vi "AutoStates.vi"(6 "WasHot?":bool, 8 "error in (no error)":errorcluster, 9 "SwitchToLowGear?":bool, 10 "AutoMode":T1, 11 "AutoState":T2) -> (0 "error out":errorcluster, 4 "Hot?":bool)   [LabVIEW 2013]
uses:
  AutoStates.ctl
  AutoMode.ctl
  DoubleSolenoidAction.ctl
  SingleSolenoidAction.ctl
  ServoAction.ctl
  RollerAction.ctl
  CollectorWrapAction.ctl
  SonarAction.ctl
  AutoAlignMode.ctl
  TankDriveAction.ctl
  ShooterWrapperAction.ctl
panel:
  out "ElapsedTime":u32
  in  "RotateWait":u32=300
  in  "RotateMotorInput":dbl=0.7
  out "RaiseArmTimedOut":bool
  in  "CollectorArmSpeed":dbl=1.0 format="%#_13g"
  in  "RaiseArmTimeout":u32=800
  in  "LowerArmTimeout":u32=800
  in  "PreRaiseArmWait":u32=500
  in  "PreShootWait":u32
  in  "StartShootTime":u32=4500
  out "DriveTimeOut":bool
  in  "MaxMotorChangeBackward":dbl=0.025
  in  "MaxMotorChangeForward":dbl=0.05
  in  "DefaultMotorInput":dbl=0.7
  in  "SlowdownDistance":dbl=24.0 format="%#_13g"
  in  "BrakeDistance":dbl=6.0 format="%#_13g"
  in  "FarShotDistance":dbl=150.0 format="%#_13g"
  in  "CloseShotDistance":dbl=36.0 format="%#_13g"
  in  "FarShotMinTime":u32=1000
  in  "CloseShotMinTime":u32=2000
  in  "FarShotTimeout":u32=4000
  in  "CloseShotTimeout":u32=4000
  in  "RaiseServoAngle":i32=100
  out "LowerArmTimedOut":bool
  in  "PreCollectWait":u32=400
  out "HotGoalTimedOut?":bool
  in  "CheckHotGoalTimeout":u32=1000
  in  "ServoInitAngle":i32=140
  # "ARM"
  # "HOT GOAL"
  # "SERVO"
  # "OUTPUT"
  # "SHOOT"
  # "ROTATE"
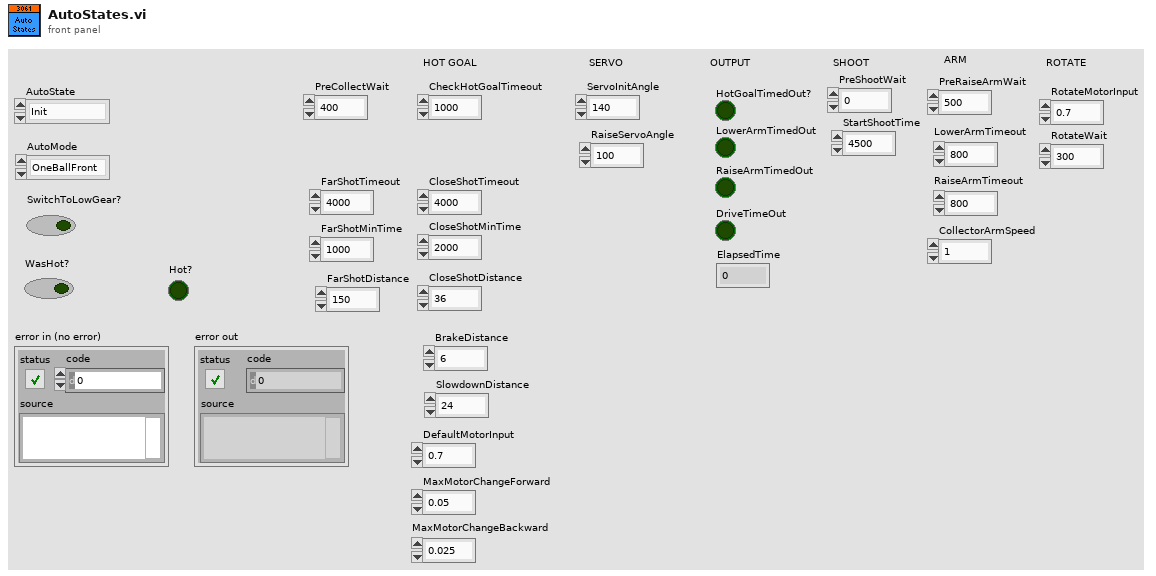
[diagram p1: front panel]
types:
  T1 = typedef "AutoMode.ctl" = enum16{"OneBallFront", "OneBallCollector", "TwoBallNormal", "TwoBallHot"}
  T2 = typedef "AutoStates.ctl" = enum16{"Init", "LowerArm", "CheckGoal", "Collect", "StopCollect", "RaiseServo", "Drive", "Wait", "ShootCollectorUp", "RaiseArm", "ShootCollectorDown", "Rotate1", "Rotate2", "Stop"}
  T3 = typedef "ServoAction.ctl" = enum16{"Init", "SetAngle", "GetAngle", "Lower", "Raise", "Disable"}
  T4 = typedef "DoubleSolenoidAction.ctl" = enum16{"Init", "Middle", "In", "Out"}
  T5 = typedef "SingleSolenoidAction.ctl" = enum16{"Init", "SetState", "Disable"}
  T6 = typedef "RollerAction.ctl" = enum16{"Init", "Off", "Forward", "Reverse"}
  T7 = typedef "CollectorWrapAction.ctl" = enum16{"PreCollect", "Collect", "Stop"}
  T8 = typedef "TankDriveAction.ctl" = enum16{"Init", "LinearDrive", "SetValue", "Disable"}
  T9 = typedef "AutoAlignMode.ctl" = enum16{"Fullspeed", "Linear"}
  T10 = typedef "SonarAction.ctl" = enum16{"Init", "ReadValue", "Disable"}
  T11 = typedef "ShooterWrapperAction.ctl" = enum16{"Init", "CollectorDown", "CollectorUp"}
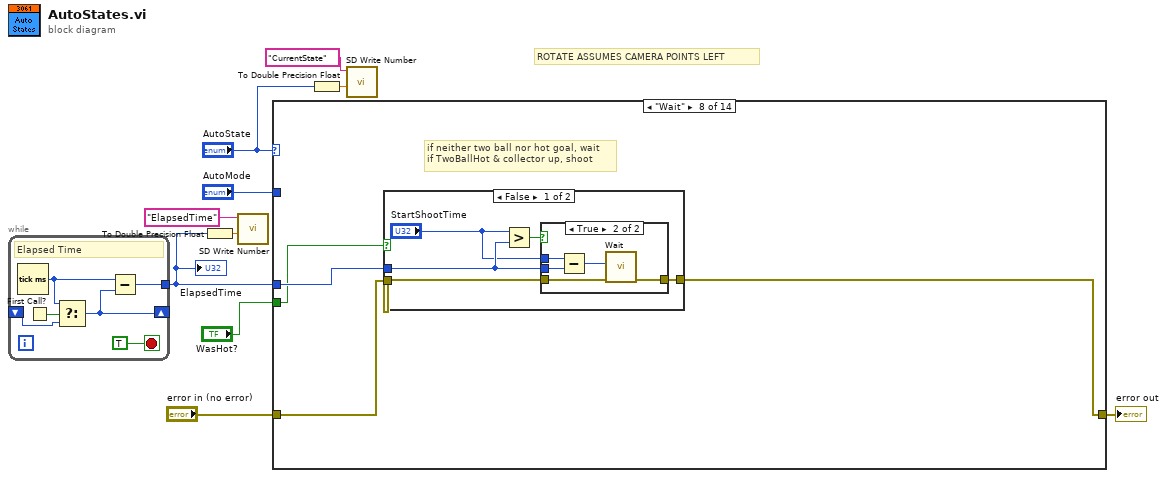
[diagram p0: block diagram]
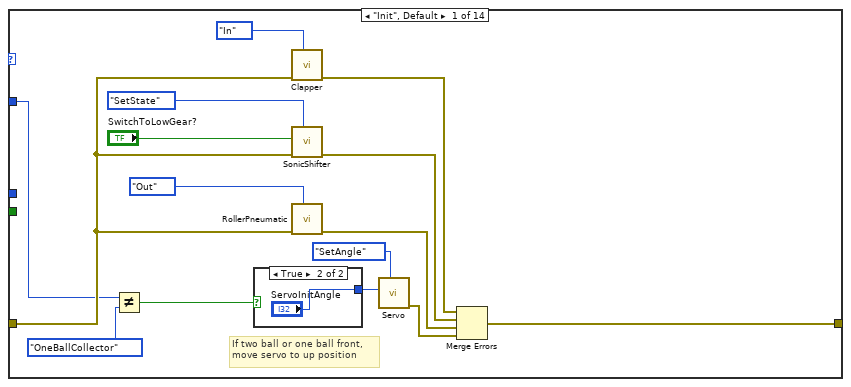
[diagram p2: hidden frame]
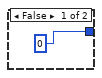
[diagram p3: hidden frame]
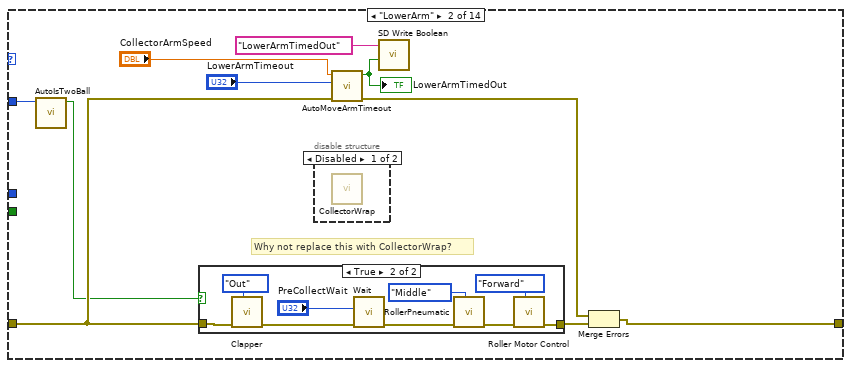
[diagram p4: hidden frame]
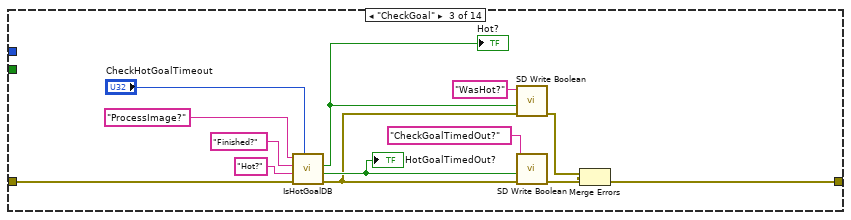
[diagram p7: hidden frame]
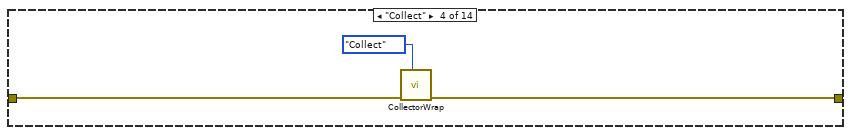
[diagram p8: hidden frame]
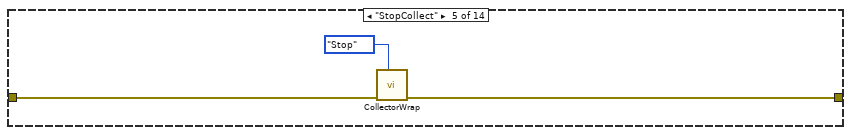
[diagram p9: hidden frame]
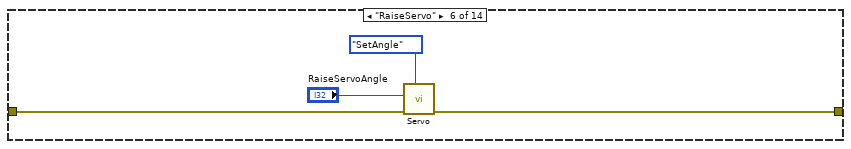
[diagram p10: hidden frame]
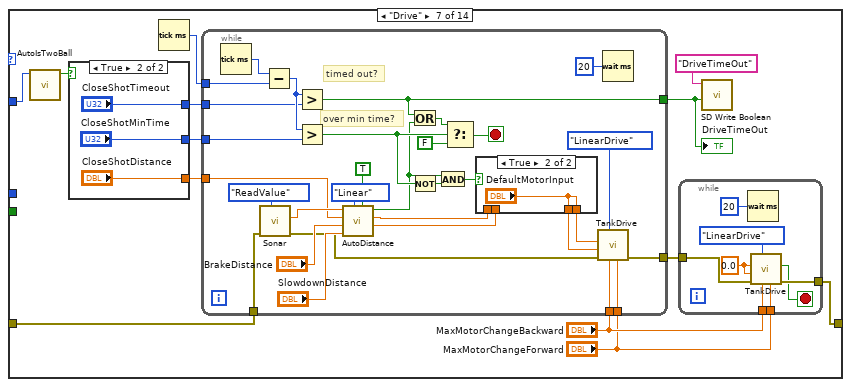
[diagram p11: hidden frame]
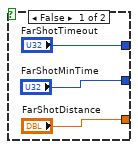
[diagram p13: hidden frame]
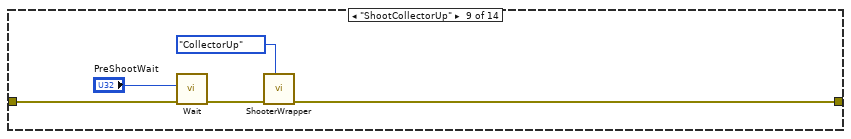
[diagram p16: hidden frame]
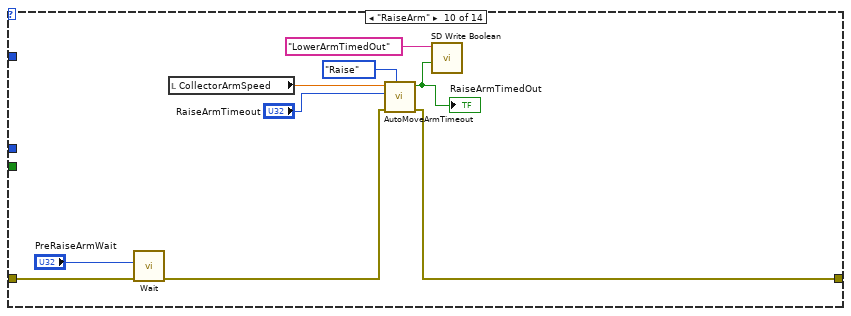
[diagram p17: hidden frame]
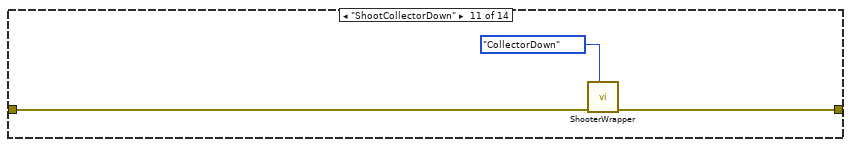
[diagram p18: hidden frame]
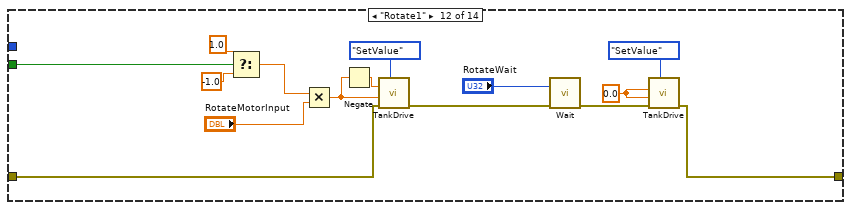
[diagram p19: hidden frame]
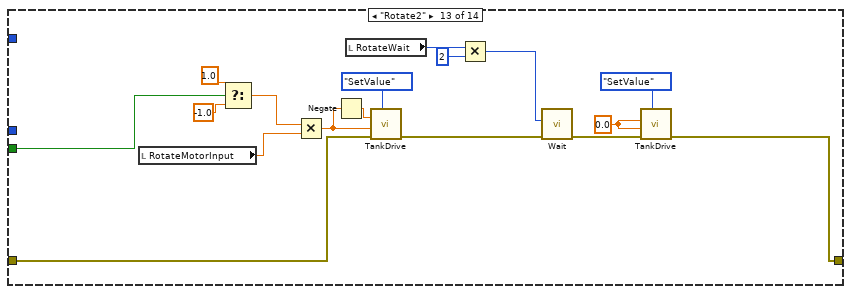
[diagram p20: hidden frame]
diagram:
  # "ROTATE ASSUMES CAMERA POINTS LEFT"
  n1 = while {
    shift-right: [w12] -> _
    shift-left: _ -> [w14]
    tunnel: [w11] -> w1
    stop <- TRUE stop-if-true
    # "Elapsed Time"
    n2 = Tick Count (ms)() -> (millisecond timer value=w13:u32)
    n3 = First Call?() -> (First Call?: T/F=w16:bool)
    n4 = Select(t=w13, s=w16, f=w14) -> (s? t:f=w12:u32)
    n5 = Subtract(x=w13, y=w12) -> (x-y=w11:u32)
  }
  "ElapsedTime" <- w1
  n6 = To Double Precision Float(number=w1) -> (double precision float=w2:dbl)
  n7 = call <vilib>:"SD Write Number.vi"("Numeric"=w2, "Name"="ElapsedTime") -> ()  [unwired: 8 in, 2 out]
  n8 = case shown="\"Wait\"" "AutoState" {
    tunnel: "AutoMode" -> [w26 w37 _ _ _ _ w89 _ _ _ _ _ _ _]
    tunnel: [w28 w41 w55 w67 w70 w74 w78 w139 w154 w161 w170 w171 w187 w203] -> w8
    tunnel: "error in (no error)" -> [w27 w42 w61 w68 w71 w73 w83 w140 w158 w166 w168 w172 w186 w204]
    tunnel: w1 -> [_ _ _ _ _ _ _ w141 _ _ _ _ _ _]
    tunnel: "WasHot?" -> [_ _ _ _ _ _ _ w138 _ _ _ w173 w188 _]
    frame "Init", Default {
      # "If two ball or one ball front, \nmove servo to up position"
      n9 = Not Equal?(x=w26, y=AutoMode."OneBallCollector") -> (x != y?=w18:bool)
      n10 = case shown="True" w18 {
        tunnel: [0 "ServoInitAngle"] -> w24
        frame False {
        }
        frame True {
        }
      }
      n11 = call "Clapper.vi"("State"=DoubleSolenoidAction."In", "Error in"=w27) -> ("Error out"=w19:errorcluster)  [unwired: 9 in]
      n12 = call "SonicShifter.vi"("Action"=SingleSolenoidAction."SetState", "error in (no error)"=w27, "Actuate?"="SwitchToLowGear?") -> ("error out"=w20:errorcluster)  [unwired: 8 in]
      n13 = call "RollerPneumatic.vi"("State"=DoubleSolenoidAction."Out", "Error in"=w27) -> ("Error out"=w21:errorcluster)  [unwired: 9 in]
      n14 = call "Servo.vi"("Action"=ServoAction."SetAngle", "Angle (deg)"=w24) -> ("error out"=w22:errorcluster)  [unwired: 8 in, 1 out]
      n15 = Merge Errors(w19, w20, w21, w22) -> (w28:errorcluster)
    }
    frame "LowerArm" {
      # "Why not replace this with CollectorWrap?"
      n16 = call "AutoIsTwoBall.vi"("AutoMode"=w37) -> ("IsTwoBall?"=w36:bool)  [unwired: 10 in]
      n17 = case shown="True" w36 {
        tunnel: [w44 w47] -> w40
        tunnel: w42 -> [w44 w48]
        frame False {
        }
        frame True {
          n18 = call "Clapper.vi"("State"=DoubleSolenoidAction."Out", "Error in"=w48) -> ("Error out"=w52:errorcluster)  [unwired: 9 in]
          n19 = call "Wait.vi"("error in"=w52, "milliseconds to wait"="PreCollectWait") -> ("error out"=w50:errorcluster)  [unwired: 9 in]
          n20 = call "RollerPneumatic.vi"("State"=DoubleSolenoidAction."Middle", "Error in"=w50) -> ("Error out"=w53:errorcluster)  [unwired: 9 in]
          n21 = call "Roller Motor Control.vi"("Action"=RollerAction."Forward", "Error in"=w53) -> ("Error out"=w47:errorcluster)  [unwired: 9 in]
        }
      }
      n22 = disable-structure shown="Disabled" {
        frame Disabled {
          n23 = call "CollectorWrap.vi"() -> ()  [unwired: 11 in, 1 out]
        }
        frame Enabled {
        }
      }
      n24 = call "AutoMoveArmTimeout.vi"("error in (no error)"=w42, "Timeout"="LowerArmTimeout", "CollectorArmSpeed"="CollectorArmSpeed") -> ("error out"=w39:errorcluster, "TimedOut?"=w38:bool)  [unwired: 7 in]
      "LowerArmTimedOut" <- w38
      n25 = call <vilib>:"SD Write Boolean.vi"("Boolean"=w38, "Name"="LowerArmTimedOut") -> ()  [unwired: 8 in, 2 out]
      n26 = Merge Errors(w39, w40) -> (w41:errorcluster)
    }
    frame "CheckGoal" {
      n27 = call "IsHotGoalDB.vi"("Timeout (ms)"="CheckHotGoalTimeout", "error in"=w61, "DBHot?"="Hot?", "DBFinished?"="Finished?", "DBStart"="ProcessImage?") -> ("error out"=w60:errorcluster, "TimedOut?"=w65:bool, "Hot?"=w54:bool)  [unwired: 4 in]
      "HotGoalTimedOut?" <- w65
      "Hot?" <- w54
      n28 = call <vilib>:"SD Write Boolean.vi"("error in"=w60, "Boolean"=w54, "Name"="WasHot?") -> ("error out"=w62:errorcluster)  [unwired: 7 in, 1 out]
      n29 = call <vilib>:"SD Write Boolean.vi"("error in"=w60, "Boolean"=w65, "Name"="CheckGoalTimedOut?") -> ("error out"=w63:errorcluster)  [unwired: 7 in, 1 out]
      n30 = Merge Errors(w62, w63) -> (w55:errorcluster)
    }
    frame "Collect" {
      n31 = call "CollectorWrap.vi"("Action"=CollectorWrapAction."Collect", "error in"=w68) -> ("error out"=w67:errorcluster)  [unwired: 9 in]
    }
    frame "StopCollect" {
      n32 = call "CollectorWrap.vi"("Action"=CollectorWrapAction."Stop", "error in"=w71) -> ("error out"=w70:errorcluster)  [unwired: 9 in]
    }
    frame "RaiseServo" {
      n33 = call "Servo.vi"("Action"=ServoAction."SetAngle", "error in (no error)"=w73, "Angle (deg)"="RaiseServoAngle") -> ("error out"=w74:errorcluster)  [unwired: 7 in, 1 out]
    }
    frame "Drive" {
      n34 = call "AutoIsTwoBall.vi"("AutoMode"=w89) -> ("IsTwoBall?"=w88:bool)  [unwired: 10 in]
      n35 = case shown="True" w88 {
        tunnel: ["FarShotTimeout" "CloseShotTimeout"] -> w86
        tunnel: ["FarShotMinTime" "CloseShotMinTime"] -> w85
        tunnel: ["FarShotDistance" "CloseShotDistance"] -> w84
        frame False {
        }
        frame True {
        }
      }
      n36 = Tick Count (ms)() -> (millisecond timer value=w87:u32)
      n37 = while {
        tunnel: w87 -> [w127]
        tunnel: w86 -> [w125]
        tunnel: w85 -> [w124]
        tunnel: w84 -> [w119]
        tunnel: w83 -> [w123]
        tunnel: [w115] -> w77
        tunnel: "MaxMotorChangeForward" -> [w101]
        tunnel: "MaxMotorChangeBackward" -> [w100]
        tunnel: [w99] -> w82
        stop <- w111 stop-if-true
        # "over min time?"
        # "timed out?"
        n38 = Tick Count (ms)() -> (millisecond timer value=w128:u32)
        n39 = call "Sonar.vi"("Action"=SonarAction."ReadValue", "error in (no error)"=w123) -> ("error out"=w103:errorcluster, "distance"=w122:dbl)  [unwired: 8 in]
        n40 = Subtract(x=w128, y=w127) -> (x-y=w126:u32)
        n41 = Greater?(x=w126, y=w125) -> (0:w115:bool)
        n42 = Greater?(x=w126, y=w124) -> (0:w113:bool)
        n43 = call "AutoDistance.vi"("Auto"=TRUE, "Mode"=AutoAlignMode."Linear", "Slowdown"="SlowdownDistance", "Brake"="BrakeDistance", "DesiredDistance"=w119, "CurrentDistance"=w122) -> ("TankDriveRight"=w106:dbl, "TankDriveLeft"=w107:dbl, "Finished"=w109:bool)  [unwired: 3 in]
        n44 = Or(x=w115, y=w109) -> (x .or. y?=w114:bool)
        n45 = Not(x=w113) -> (.not. x?=w110:bool)
        n46 = And(x=w109, y=w110) -> (x .and. y?=w108:bool)
        n47 = Select(t=w114, s=w113, f=FALSE) -> (s? t:f=w111:bool)
        n48 = case shown="True" w108 {
          tunnel: w107 -> [w129 _]
          tunnel: w106 -> [w130 _]
          tunnel: [w130 "DefaultMotorInput"] -> w104
          tunnel: [w129 "DefaultMotorInput"] -> w105
          frame False {
          }
          frame True {
          }
        }
        n49 = call "TankDrive.vi"("MaxMotorChangeForward"=w101, "MaxMotorChangeBackwrad"=w100, "DriveAction"=TankDriveAction."LinearDrive", "error in (no error)"=w103, "RightDesired"=w104, "LeftDesired"=w105) -> ("error out"=w99:errorcluster)  [unwired: 4 in, 1 out]
        n50 = Wait (ms)(milliseconds to wait=u32 20) -> ()  [unwired: 1 out]
      }
      "DriveTimeOut" <- w77
      n51 = while {
        tunnel: w82 -> [w97]
        tunnel: [w96] -> w78
        tunnel: "MaxMotorChangeForward" -> [w91]
        tunnel: "MaxMotorChangeBackward" -> [w90]
        stop <- w92 stop-if-true
        w95 = 0.0 ("LeftDesired")
        n52 = Wait (ms)(milliseconds to wait=u32 20) -> ()  [unwired: 1 out]
        n53 = call "TankDrive.vi"("MaxMotorChangeForward"=w91, "MaxMotorChangeBackwrad"=w90, "DriveAction"=TankDriveAction."LinearDrive", "error in (no error)"=w97, "RightDesired"=w95, "LeftDesired"=w95) -> ("error out"=w96:errorcluster, "InRange?"=w92:bool)  [unwired: 4 in]
      }
      n54 = call <vilib>:"SD Write Boolean.vi"("Boolean"=w77, "Name"="DriveTimeOut") -> ()  [unwired: 8 in, 2 out]
    }
    frame "Wait" {
      # "if neither two ball nor hot goal, wait\nif TwoBallHot & collector up, shoot"
      n55 = case shown="False" w138 {
        tunnel: w141 -> [w145 _]
        tunnel: w140 -> [w143 w153]
        tunnel: [w142 w153] -> w139
        frame False {
          n56 = Greater?(x="StartShootTime", y=w145) -> (0:w146:bool)
          n57 = case shown="True" w146 {
            tunnel: w145 -> [_ w151]
            tunnel: "StartShootTime" -> [_ w150]
            tunnel: w143 -> [w147 w149]
            tunnel: [w147 w148] -> w142
            frame False {
            }
            frame True {
              n58 = Subtract(x=w150, y=w151) -> (x-y=w152:u32)
              n59 = call "Wait.vi"("error in"=w149, "milliseconds to wait"=w152) -> ("error out"=w148:errorcluster)  [unwired: 9 in]
            }
          }
        }
        frame True {
        }
      }
    }
    frame "ShootCollectorUp" {
      n60 = call "Wait.vi"("error in"=w158, "milliseconds to wait"="PreShootWait") -> ("error out"=w156:errorcluster)  [unwired: 9 in]
      n61 = call "ShooterWrapper.vi"("Action"=ShooterWrapperAction."CollectorUp", "error in"=w156) -> ("error out"=w154:errorcluster)  [unwired: 8 in]
    }
    frame "RaiseArm" {
      n62 = call "Wait.vi"("error in"=w166, "milliseconds to wait"="PreRaiseArmWait") -> ("error out"=w165:errorcluster)  [unwired: 9 in]
      n63 = local read "CollectorArmSpeed"() -> (w159:dbl)
      n64 = call "AutoMoveArmTimeout.vi"("Action"=enum16{"Lower", "Raise"}."Raise", "error in (no error)"=w165, "Timeout"="RaiseArmTimeout", "CollectorArmSpeed"=w159) -> ("error out"=w161:errorcluster, "TimedOut?"=w160:bool)  [unwired: 6 in]
      "RaiseArmTimedOut" <- w160
      n65 = call <vilib>:"SD Write Boolean.vi"("Boolean"=w160, "Name"="LowerArmTimedOut") -> ()  [unwired: 8 in, 2 out]
    }
    frame "ShootCollectorDown" {
      n66 = call "ShooterWrapper.vi"("Action"=ShooterWrapperAction."CollectorDown", "error in"=w168) -> ("error out"=w170:errorcluster)  [unwired: 8 in]
    }
    frame "Rotate1" {
      w177 = 0.0
      n67 = Select(t=1.0, s=w173, f=-1.0) -> (s? t:f=w184:dbl)
      n68 = Multiply(x=w184, y="RotateMotorInput") -> (x*y=w182:dbl)
      n69 = Negate(x=w182) -> (-x=w181:dbl)
      n70 = call "TankDrive.vi"("DriveAction"=TankDriveAction."SetValue", "error in (no error)"=w172, "RightDesired"=w182, "LeftDesired"=w181) -> ("error out"=w179:errorcluster)  [unwired: 6 in, 1 out]
      n71 = call "Wait.vi"("error in"=w179, "milliseconds to wait"="RotateWait") -> ("error out"=w178:errorcluster)  [unwired: 9 in]
      n72 = call "TankDrive.vi"("DriveAction"=TankDriveAction."SetValue", "error in (no error)"=w178, "RightDesired"=w177, "LeftDesired"=w177) -> ("error out"=w171:errorcluster)  [unwired: 6 in, 1 out]
    }
    frame "Rotate2" {
      w194 = 0.0
      n73 = local read "RotateMotorInput"() -> (w192:dbl)
      n74 = Select(t=1.0, s=w188, f=-1.0) -> (s? t:f=w201:dbl)
      n75 = Multiply(x=w201, y=w192) -> (x*y=w199:dbl)
      n76 = Negate(x=w199) -> (-x=w198:dbl)
      n77 = local read "RotateWait"() -> (w191:u32)
      n78 = call "TankDrive.vi"("DriveAction"=TankDriveAction."SetValue", "error in (no error)"=w186, "RightDesired"=w199, "LeftDesired"=w198) -> ("error out"=w196:errorcluster)  [unwired: 6 in, 1 out]
      n79 = Multiply(x=w191, y=u32 2) -> (x*y=w189:u32)
      n80 = call "Wait.vi"("error in"=w196, "milliseconds to wait"=w189) -> ("error out"=w195:errorcluster)  [unwired: 9 in]
      n81 = call "TankDrive.vi"("DriveAction"=TankDriveAction."SetValue", "error in (no error)"=w195, "RightDesired"=w194, "LeftDesired"=w194) -> ("error out"=w187:errorcluster)  [unwired: 6 in, 1 out]
    }
    frame "Stop" {
      n82 = call "Servo.vi"("Action"=ServoAction."SetAngle", "error in (no error)"=w204, "Angle (deg)"=0) -> ("error out"=w209:errorcluster)  [unwired: 7 in, 1 out]
      n83 = call "SonicShifter.vi"("Action"=SingleSolenoidAction."SetState", "error in (no error)"=w209, "Actuate?"=FALSE) -> ("error out"=w203:errorcluster)  [unwired: 8 in]
    }
  }
  "error out" <- w8
  n84 = To Double Precision Float(number="AutoState") -> (double precision float=w6:dbl)
  n85 = call <vilib>:"SD Write Number.vi"("Numeric"=w6, "Name"="CurrentState") -> ()  [unwired: 8 in, 2 out]
